vi "Wrapper_closeAllSpectrometers.vi"(1 "Wrapper In":u32) -> (0 "Wrapper Out":u32)   [LabVIEW 2017]
uses:
  OmniDriver32.dll
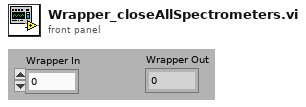
[diagram p1: front panel]
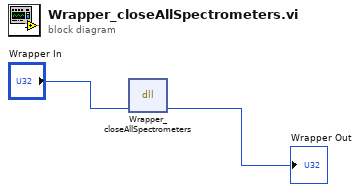
[diagram p0: block diagram]
diagram:
  n1 = dll-call lib="OmniDriver32.dll" fn="Wrapper_closeAllSpectrometers" label="Wrapper.closeAllSpectrometers"("Wrapper"="Wrapper In") -> ("Wrapper"=→"Wrapper Out":u32)  [unwired: 3 in, 3 out]
